vi "OL_control.vi"(8 "Motor_index":i32[](array[numeric])=[3, 6, 9, 12, 2, 7, 8, 13, 4, 5, 10, 11, 1, 14], 11 "goal_Tensions":dbl[](array[numeric])) -> (3 "can_Current":dbl[](array[numeric]))   [LabVIEW 2024]
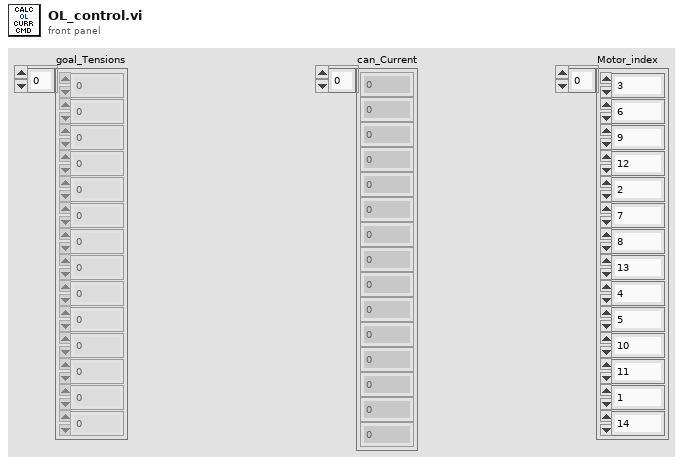
[diagram p1: front panel]
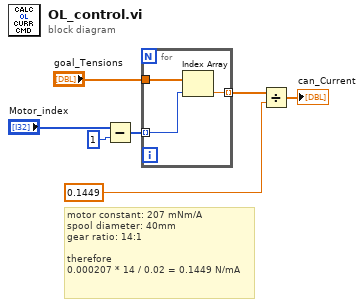
[diagram p0: block diagram]
diagram:
  # "motor constant: 207 mNm/A\nspool diameter: 40mm\ngear ratio: 14:1\n\ntherefore\n0.000207 * 14 / 0.02 = 0.1449 N/mA"
  n1 = Subtract(x="Motor_index", y=1) -> (x-y=w3:i32[])
  n2 = for {
    tunnel: w3 -> [w10] mode=indexing
    tunnel: "goal_Tensions" -> [w9]
    tunnel: [w8] -> w1 mode=indexing
    n3 = Index Array(array=w9, index=w10) -> (element=w8:dbl)
  }
  n4 = Divide(x=w1, y=0.1449) -> (x/y=→"can_Current":dbl[])
